vi "HoppingStep(Nonlinear-XZOnly).vi"() -> ()   [LabVIEW 2014]
uses:
  <vilib>/Platform/TimedLoop/XDataNode/timing_clust.ctl
  <vilib>/Platform/TimedLoop/XDataNode/nitl_modes.ctl
  <vilib>/Platform/TimedLoop/XDataNode/wakeup.ctl
  <vilib>/rvi/Emulation/niFpgaGetClockAttributes.vi
  <vilib>/rvi/Emulation/niFpgaSctlEmulationGetInTimedLoop.vi
  <vilib>/rvi/Emulation/niFpgaEmulationReportErrorSimple.vi
  <vilib>/rvi/eio/common/nirviEmuTemplateMethod_errors.vi
  <vilib>/rvi/Emulation/niFpgaCriticalErrorInLSC.vi
  <vilib>/rvi/interface/RandomDataEmulation/niFpgaRandomDataHandleErrors.vi
  <vilib>/rvi/Emulation/niFpgaProcessEmulError.vi
  <vilib>/eio/EIONode/EIONode.xnode
  <vilib>/Platform/TimedLoop/XDataNode/XDataNode.xnode
  <vilib>/rvi/DataTransferAndStorage/Container/XNode/niFpgaContainer.xnode
  <vilib>/rvi/interface/RandomDataEmulation/nirviRandomDataFpgaReadWriteTemplate.vi
  <vilib>/Platform/TimedLoop/XDataNode/XDNodeRunTimeDep.lvlib
panel:
  out "ZRealPos":i16
  in  "RelativeWithdraw":i16
  out "Waveform Chart":i32(graph)
  in  "stop":bool
  out "Z":i32(graph)
  in  "ZOffset":i16
  in  "XOffset":i16
  in  "XNum":i16
  in  "XStepIndex":i16
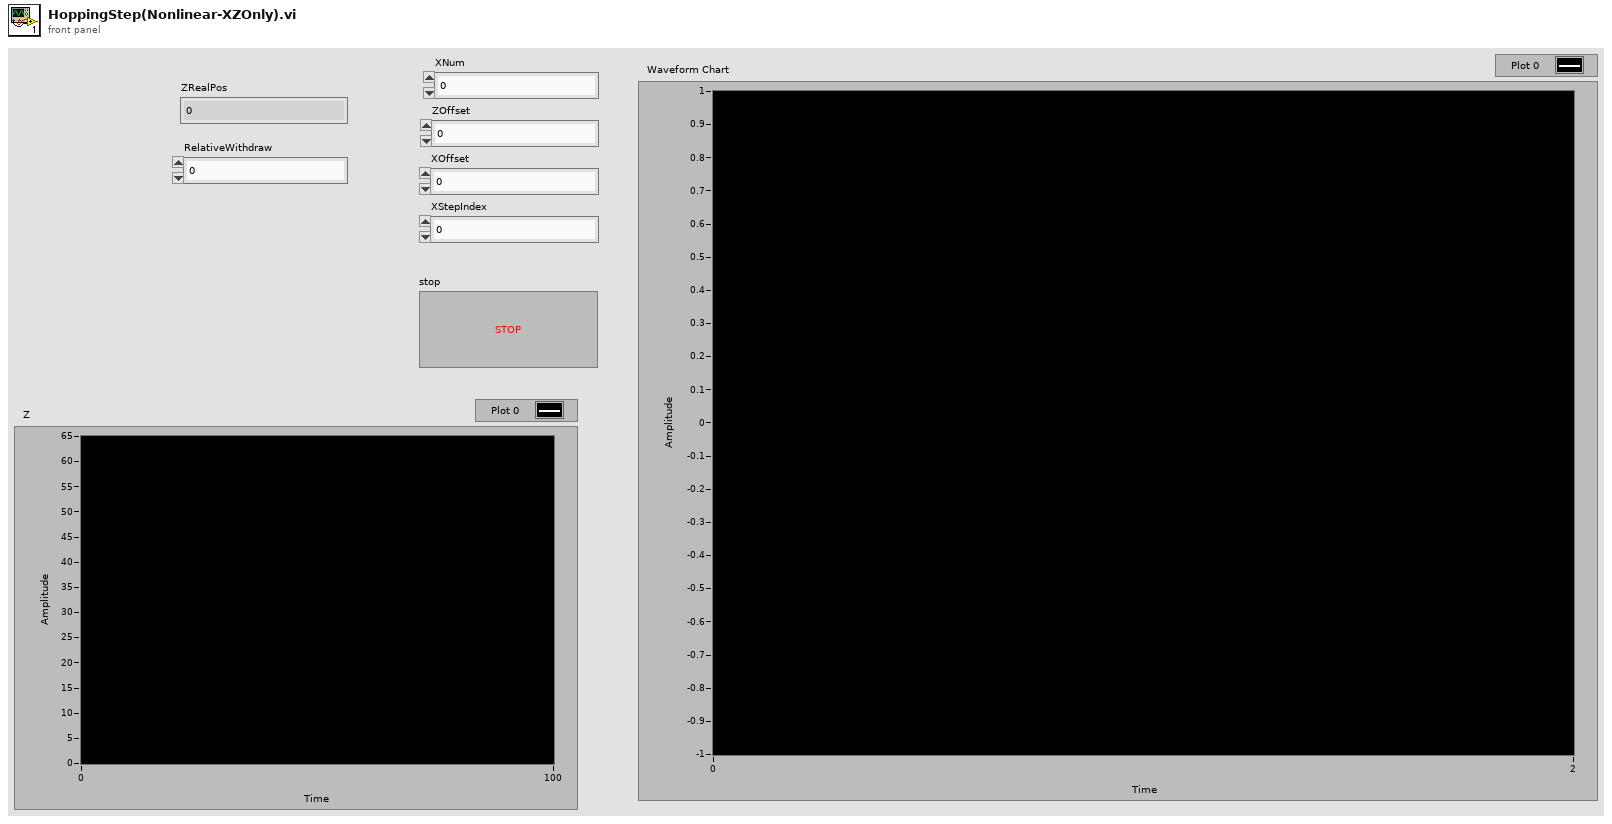
[diagram p1: front panel]
types:
  T1 = typedef "XDNodeRunTimeDep.lvlib/timing_clust.ctl" = cluster{"Expected End [f-1]":u64, "Actual End [f-1]":u64, "Finished Late? [f-1]":bool, "Expected End [i-1]":u64, "Actual End [i-1]":u64, "Finished Late? [i-1]":bool, "Expected Start [i]":u64, "Actual Start [i]":u64, "Expected Start [f]":u64, "Actual Start [f]":u64, "Source Name":string, "Structure Name":string, "Period":i64, "Deadline":i64, "Offset":i64, "Start":i64, "Priority":i32, "Timeout":i32, "Mode":T2, "Wakeup Reason":T3, "Error":errorcluster, "Source Type":string, "Secondary Source Type":string, "Global End Time":u64, "Global Start Time":u64, "Frame Duration":u64, "Iteration Duration":u64, "Assigned CPU":i32, "I/O Scan Engine Mode":u32}
  T2 = typedef "XDNodeRunTimeDep.lvlib/nitl_modes.ctl" = enum32{"No Change", "Process missed periods, maintain original phase", "Discard missed periods, maintain original phase", "Process missed periods, ignore original phase", "Discard missed periods, ignore original phase"}
  T3 = typedef "XDNodeRunTimeDep.lvlib/wakeup.ctl" = enum32{"Normal", "Aborted", "Asynchronous wakeup", "Timing source error", "Timed loop error", "Timeout"}
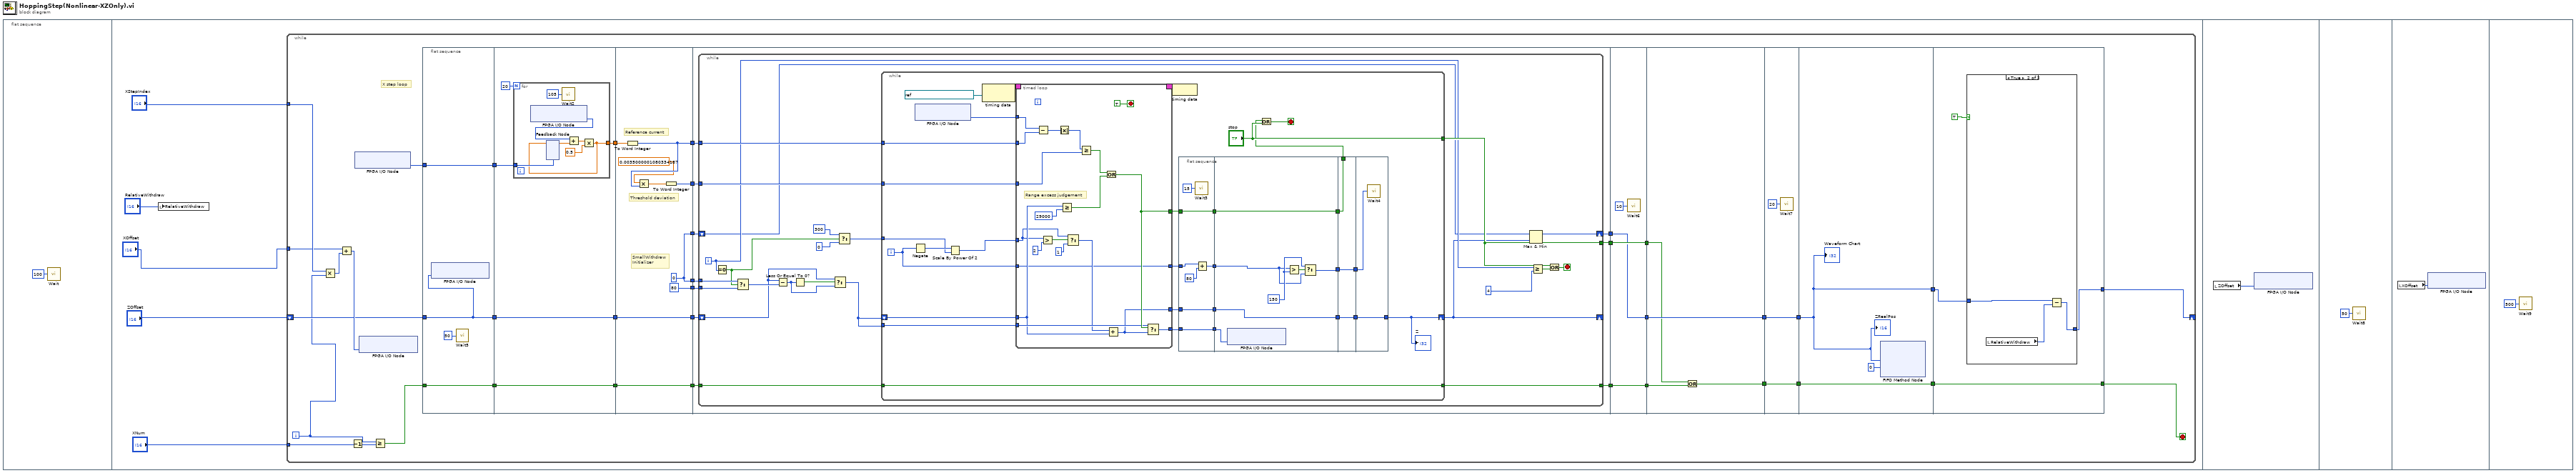
[diagram p0: block diagram]
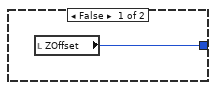
[diagram p2: hidden frame]
diagram:
  n1 = flat-sequence {
    frame #0 {
      n2 = call "Wait"("Count(mSec)"=u32 100 ("Count(uSec)")) -> ()  [unwired: 1 out]
    }
    frame #1 {
      n3 = local write "RelativeWithdraw"("RelativeWithdraw") -> ()
      n4 = while {
        tunnel: "XNum" -> [w19]
        tunnel: "XStepIndex" -> [w20]
        shift-right: [w7] -> _
        shift-left: "ZOffset" -> [w21]
        tunnel: "XOffset" -> [w10]
        i -> [w11]
        stop <- w30 stop-if-true
        # "X step loop"
        n5 = Multiply(x=w20, y=w11) -> (x*y=w25:i32)
        n6 = Add(x=w10, y=w25) -> (x+y=w26:i32)
        n7 = Decrement(x=w19) -> (x-1=w18:i16)
        n8 = xnode "FPGA I/O Node"() -> ("Connector0/AI1"=w37:i16)  [unwired: 1 in, 1 out]
        n9 = xnode "FPGA I/O Node"("Connector0/AO2"=w26) -> ()  [unwired: 1 in, 1 out]
        n10 = Greater Or Equal?(x=w11, y=w18) -> (x >= y?=w17:bool)
        n11 = flat-sequence {
          tunnel: [w46] -> w42
          tunnel: w37 -> [w46]
          tunnel: [w45] -> w27
          tunnel: w21 -> [w45]
          tunnel: w17 -> [w44]
          tunnel: [w44] -> w16
          tunnel: w42 -> [w52]
          tunnel: [w50] -> w41
          tunnel: [w49] -> w28
          tunnel: w27 -> [w49]
          tunnel: w16 -> [w48]
          tunnel: [w48] -> w15
          tunnel: [w62] -> w43
          tunnel: w41 -> [w68]
          tunnel: [w67] -> w40
          tunnel: [w64] -> w39
          tunnel: [i16 80] -> w29
          tunnel: w28 -> [w62]
          tunnel: [w61] -> w24
          tunnel: [w61] -> w23
          tunnel: w15 -> [w60]
          tunnel: [w60] -> w14
          tunnel: w39 -> [w76]
          tunnel: w40 -> [w77]
          tunnel: w43 -> [w78]
          tunnel: [w75] -> w33
          tunnel: w29 -> [w74]
          tunnel: w24 -> [w73]
          tunnel: w23 -> [w72]
          tunnel: [w71] -> w22
          tunnel: w14 -> [w70]
          tunnel: [w69] -> w12
          tunnel: [w178] -> w38
          tunnel: [w179] -> w34
          tunnel: w33 -> [w179]
          tunnel: w22 -> [w178]
          tunnel: [w177] -> w13
          tunnel: w12 -> [w177]
          tunnel: w38 -> [w184]
          tunnel: [w184] -> w36
          tunnel: w34 -> [w183]
          tunnel: [w182] -> w31
          tunnel: w13 -> [w181]
          tunnel: w36 -> [w186]
          tunnel: [w186] -> w35
          tunnel: [w185] -> w32
          tunnel: w31 -> [w185]
          tunnel: w35 -> [w188]
          tunnel: w32 -> [w189]
          tunnel: [w189] -> w9
          tunnel: [w188] -> w8
          tunnel: [w192] -> w7
          tunnel: [w194] -> w30
          tunnel: w9 -> [w194]
          tunnel: w8 -> [w191]
          frame #0 {
            n12 = xnode "FPGA I/O Node"("Connector0/AO0"=w45) -> ()  [unwired: 1 in, 1 out]
            n13 = call "Wait5"("Count(uSec)"=u32 50) -> ()  [unwired: 1 out]
          }
          frame #1 {
            n14 = for {
              N: 20 -> [_]
              tunnel: w52 -> [w58]
              tunnel: [w53] -> w50
              n15 = xnode "FPGA I/O Node"() -> ("Connector0/AI1"=w56:i16)  [unwired: 1 in, 1 out]
              n16 = feedback #1(w58) -> (w57:sgl)
              n17 = call "Wait2"("Count(uSec)"=u32 105) -> ()  [unwired: 1 out]
              n18 = Add(x=w56, y=w57) -> (x+y=w55:sgl)
              n19 = Multiply(x=w55, y=sgl 0.5) -> (x*y=w53:sgl)
              n20 = feedback-in #1(w53) -> ()
            }
          }
          frame #2 {
            w61 = i16 0
            # "SmallWithdraw\nInitializer"
            # "Threshold deviation"
            # "Reference current"
            n21 = To Word Integer(number=w68) -> (16bit integer=w67:i16)
            n22 = Multiply(x=sgl 0.0035, y=w67) -> (x*y=w65:sgl)
            n23 = To Word Integer(number=w65) -> (16bit integer=w64:i16)
          }
          frame #3 {
            n24 = while {
              tunnel: w77 -> [w101]
              tunnel: w76 -> [w100]
              tunnel: [w97] -> w75
              tunnel: w74 -> [w95]
              shift-right: [w87] -> _
              shift-left: w78 -> [w92]
              tunnel: w73 -> [w89]
              shift-right: [w86] -> w71
              shift-left: w72 -> [w88]
              tunnel: w70 -> [w81]
              tunnel: [w80] -> w69
              i -> [w96]
              stop <- w99 stop-if-true
              n25 = Equal To 0?(x=w96) -> (x = 0?=w85:bool)
              n26 = Select(t=w89, s=w85, f=w95) -> (s? t:f=w94:i16)
              n27 = Subtract(x=w92, y=w94) -> (x-y=w91:i32)
              n28 = Less Or Equal To 0?(x=w91) -> (x <= 0?=w93:bool)
              n29 = Select(t=w92, s=w93, f=w91) -> (s? t:f=w90:i32)
              n30 = Select(t=i16 300, s=w85, f=i16 0) -> (s? t:f=w82:i16)
              n31 = while {
                tunnel: w101 -> [w124]
                tunnel: w100 -> [w126]
                tunnel: ["stop"] -> w97
                shift-right: [w115] -> w87
                shift-left: w90 -> [w121]
                tunnel: w90 -> [w118]
                tunnel: w82 -> [w105]
                tunnel: w81 -> [w102]
                tunnel: [w102] -> w80
                i -> [w103]
                stop <- w128 stop-if-true
                n32 = Negate(x=w103) -> (-x=w106:i32)
                n33 = xnode "FPGA I/O Node"() -> ("Connector0/AI1"=w125:i16)  [unwired: 1 in, 1 out]
                n34 = Scale By Power Of 2(n=w106, x=w105) -> (x*2^n=w104:i16)
                n35 = node-c288(refnum<k21> "40 MHz Onboard Clock" ("Source Name")) -> (w131:T1)
                n36 = timed-loop {
                  timing: w131 -> [_]
                  timing-out: [_] -> w130
                  tunnel: w124 -> [w168]
                  tunnel: w126 -> [w151]
                  tunnel: w125 -> [w169]
                  tunnel: [w164] -> w122
                  tunnel: [w163] -> w120
                  tunnel: w121 -> [w160]
                  tunnel: w118 -> [w162]
                  tunnel: [w159] -> w117
                  tunnel: w104 -> [w154]
                  tunnel: [w156] -> w107
                  tunnel: w103 -> [w156]
                  stop <- TRUE stop-if-true
                  # "Range excess judgement"
                  n37 = Subtract(x=w169, y=w168) -> (x-y=w152:i16)
                  n38 = Greater?(x=w154, y=i16 2) -> (0:w153:bool)
                  n39 = Absolute Value(x=w152) -> (abs(x)=w167:i16)
                  n40 = Greater Or Equal?(x=w160, y=i16 29000) -> (x >= y?=w165:bool)
                  n41 = Select(t=w154, s=w153, f=1) -> (s? t:f=w157:i32)
                  n42 = Greater Or Equal?(x=w167, y=w151) -> (x >= y?=w166:bool)
                  n43 = Or(x=w166, y=w165) -> (x .or. y?=w163:bool)
                  n44 = Add(x=w157, y=w160) -> (x+y=w159:i32)
                  n45 = Select(t=w162, s=w163, f=w159) -> (s? t:f=w164:i32)
                }
                n46 = node-c288(w130) -> ()
                n47 = flat-sequence {
                  tunnel: [w137] -> w123
                  tunnel: w122 -> [w137]
                  tunnel: w120 -> [w136]
                  tunnel: [w136] -> w119
                  tunnel: w117 -> [w135]
                  tunnel: [w135] -> w116
                  tunnel: [w133] -> w108
                  tunnel: w107 -> [w134]
                  tunnel: w123 -> [w143]
                  tunnel: [w145] -> w114
                  tunnel: w119 -> [w144]
                  tunnel: w116 -> [w145]
                  tunnel: [w144] -> w112
                  tunnel: [w140] -> w109
                  tunnel: w108 -> [w139]
                  tunnel: w114 -> [w148]
                  tunnel: [w148] -> w113
                  tunnel: w112 -> [w147]
                  tunnel: [w147] -> w111
                  tunnel: [w146] -> w110
                  tunnel: w109 -> [w146]
                  tunnel: w113 -> [w150]
                  tunnel: [w150] -> w115
                  tunnel: w110 -> [w149]
                  frame #0 {
                    n48 = call "Wait3"("Count(uSec)"=u32 15) -> ()  [unwired: 1 out]
                    n49 = Add(x=w134, y=80) -> (x+y=w133:i32)
                  }
                  frame #1 {
                    w141 = i16 150
                    n50 = xnode "FPGA I/O Node"("Connector0/AO0"=w143) -> ()  [unwired: 1 in, 1 out]
                    n51 = Greater?(x=w139, y=w141) -> (0:w142:bool)
                    n52 = Select(t=w141, s=w142, f=w139) -> (s? t:f=w140:i32)
                  }
                  frame #2 {
                  }
                  frame #3 {
                    n53 = call "Wait4"("Count(uSec)"=w149) -> ()  [unwired: 1 out]
                  }
                }
                n54 = Or(x=w111, y="stop") -> (x .or. y?=w128:bool)
                "Z" <- w115
              }
              n55 = Max & Min(x=w88, y=w87) -> (max(x,y)=w86:i32)  [unwired: 1 out]
              n56 = Greater Or Equal?(x=w96, y=4) -> (x >= y?=w98:bool)
              n57 = Or(x=w97, y=w98) -> (x .or. y?=w99:bool)
            }
          }
          frame #4 {
            n58 = call "Wait6"("Count(uSec)"=u32 10) -> ()  [unwired: 1 out]
          }
          frame #5 {
            n59 = Or(x=w183, y=w181) -> (x .or. y?=w182:bool)
          }
          frame #6 {
            n60 = call "Wait7"("Count(uSec)"=u32 20) -> ()  [unwired: 1 out]
          }
          frame #7 {
            n61 = xnode ("FIFO Method Node")("Element"=w188, "Timeout"=0) -> ()  [unwired: 1 in, 2 out]
            "Waveform Chart" <- w188
            "ZRealPos" <- w188
          }
          frame #8 {
            n62 = case shown="True" TRUE {
              tunnel: w191 -> [_ w198]
              tunnel: [w195 w196] -> w192
              frame False {
                n63 = local read "ZOffset"() -> (w195:i16)
              }
              frame True {
                n64 = local read "RelativeWithdraw"() -> (w197:i16)
                n65 = Subtract(x=w198, y=w197) -> (x-y=w196:i32)
              }
            }
          }
        }
      }
    }
    frame #2 {
      n66 = local read "ZOffset"() -> (w199:i16)
      n67 = xnode "FPGA I/O Node"("Connector0/AO0"=w199) -> ()  [unwired: 1 in, 1 out]
    }
    frame #3 {
      n68 = call "Wait8"("Count(uSec)"=u32 50) -> ()  [unwired: 1 out]
    }
    frame #4 {
      n69 = local read "XOffset"() -> (w201:i16)
      n70 = xnode "FPGA I/O Node"("Connector0/AO2"=w201) -> ()  [unwired: 1 in, 1 out]
    }
    frame #5 {
      n71 = call "Wait9"("Count(uSec)"=u32 500) -> ()  [unwired: 1 out]
    }
  }
